vi "Pacemaker ASIC Test_Conditon Globals.vi"() -> ()   [LabVIEW 2016]
uses:
  AET/TypeDef/Pacemaker ASIC Test_Relay Status.ctl
  AET/TypeDef/Pacemaker ASIC Test_Function.ctl
  AET/TypeDef/Pacemaker ASIC Test_Relay Which.ctl
  AET/TypeDef/Pacemaker ASIC Test_Register Mark Type.ctl
  step type.ctl
panel:
  in  "Rk_30":dbl=30000.0
  in  "R 12p5X":dbl
  in  "P 100X":dbl
  in  "PV [C]":dbl=37.0
  in  "Rs_Offset":dbl=23700.0
  in  "175k Downlink Vpp[V]":dbl=0.33
  in  "Rk_20":dbl=24222.307131117894
  in  "Step Type Name":T1=["Basic Setting", "Ibat Test", "Ib Trim Test", "Ib Vs Temp Test", "Ib Vs Vbat Test", "Vref Trim Test", "Vref Vs Temp Test", "Vref Vs Vbat Test", "Vref PSR Test", "VregD Trim Test", "VregD Vs Temp Test", "VregD Vs Vbat Test", "VregD Vs Load Test", "VregD PSR Test", "VregA Trim Test", "VregA Vs Temp Test", "VregA Vs Vbat Test", "VregA Vs Load Test", "VregA PSR Test", "Sense OS1 OS2 Trim Test", "Sense Lpf Hpf Trim Test", "Sense IBIPT Trim Test", "Sense Triangle Waveform Gain Vi Test", "Sense Triangle Waveform Gain Gainout Test", "Sense Pace Rejection Low Sensitivity Test", "Sense Pace Rejection High Sensitivity Test", "Sense Idle Noise Test", "Sense Drain Current Test", "Sense PSR Test", "Sense Pos Triangle Waveform Threshold Test", "Sense Neg Triangle Waveform Threshold Test", "Sense Delay Time 1 Test", "Sense Delay Time 2 Test", "Sense Sine2 Sensitivity Curve Test", "Sense After Sense Test", "Sense After Pace Test", "Sense CMRR Test", "Sense Input Impedance Test", "Pace Pump Efficiency Test", "Pace VH Test", "Pace Recharge Voltage Remain Test", "Pace Amp Test", "Pace Amp GB Test", "Pace Amp 200us Test", "Pace Amp 200us Vs Temp Test", "Pace Amp 200us Vs Battery Imp Test", "Pace Amp 200us Vs PW Test", "Pace Amp 200us Vs Rate Test", "Pace Pulse Width Test", "RC32k Trim Test", "RC32k Jitter Test", "RC32k Vs Vbat Test", "RC1p6k Trim Test", "RC1p6k Jitter Test", "RC1p6k Vs Vbat Test", "32k Crystal Input Under Voltage Test", "32k Crystal Turn on Time Test", "32k Crystal Freq Vs Temp Test", "32k Crystal Duty Vs Temp Test", "32k Crystal Freq Vs Vbat Test", "32k Crystal Duty Vs Vbat Test", "32k Crystal Jitter Test", "Por Power Up Test", "Porn VregD Power Up Test", "Por Power Down Test", "Por Nlsd Power Down Test", "Porn VregD Power Down Test", "Por Glitch Test", "Ant Receive Turn On Time Test", "Ant Receive Turn Off Time Test", "Ant Receive Threshold Test", "Ant Send Drain Current Test", "Ant Send Vpp Test", "ADC Dynamic Parameters Test", "ADC Lead Impedance Test", "ReedSwitch Vs Vbat Test", "Battery Load Impedance Test", "Battery Impedance Test", "Digital 1 Test", "ADC Static Parameters Test", "PR Detection Accuracy Test", "PR Detection Drop Voltage Test", "PR Detection PSR Test", "PR Detection Drain Current Test", "PR Detection Idle Noise Test", "PR Detection Deviation Test", "RC32k Clock Switch Test", "Digital 2 Test", "Register Reset", "Set Rst_Ext", "Trim", "ADC VH Test", "Sense Output Unique Test", "BandGap Setpoint Test", "32k Crystal Setpoint Test", "RC32k Input Under Voltage Test", "RC1p6k Input Under Voltage Test", "ADC Battery V1 Test", "ADC EGM Test", "Pace Average Current Test", "Sense Dynamic Performance Test", "Relay Reset", "Power OnOff", "Set 0V", "ADC Battery V2 Test", "Sense Sine Dynamic Range Test", "Sense Triangle Dynamic Range Test", "Check ASIC VVI\n", "pace gb voltage", "Test Done\n", "Step Test\n", "pace gb pluse width", "pace gb pluse frequency", "pace gb pluse interval", "sensitivity threshold", "MRI Threshold  Cal Test", "MRI Threshold Test"]
  in  "T":dbl
  in  "Reg Data":u8 format="%02x"
  in  "Reg Mark":T2=enum."TRIM_BANDGAPV"
  in  "Relay Index0":T3[](array[typedef])=[enum."CrystalOX2", enum."DtoOutput", enum."spiPXIpacePXI", enum."ADCinNC", enum."noloadcurrent", enum."IPGInputZNC", enum."ReedinDo", enum."AntLC", enum."nomeas", enum."RegDCurNC", enum."LoadRNC", enum."CurrentPumpNC", enum."CurrentSenseNC", enum."Anosignor", enum."Vnosignor", enum."bat0w", enum."currentMeas1", enum."currentMeas2", enum."CrystalOX2", enum."CrystalOX2", enum."CrystalOX2", enum."CrystalOX2", enum."CrystalOX2", enum."CrystalOX2", enum."CrystalOX2", enum."CrystalOX2", enum."CrystalOX2", enum."CrystalOX2", enum."CrystalOX2", enum."CrystalOX2", enum."CrystalOX2", enum."CrystalOX2", enum."CrystalOX2", enum."CrystalOX2", enum."CrystalOX2", enum."CrystalOX2", enum."CrystalOX2"]
  in  "Relay Default":T3[](array[typedef])=[enum."CrystalOX2", enum."DtoOutput", enum."spiPXIpacePXI", enum."ADCinNC", enum."noloadcurrent", enum."IPGInputZNC", enum."ReedinDo", enum."AntLC", enum."nomeas", enum."RegDCurNC", enum."LoadRNC", enum."CurrentPumpNC", enum."CurrentSenseNC", enum."Anosig250w", enum."Vnosig250w", enum."bat200w", enum."currentMeas1", enum."currentMeas2"]
  in  "PS [V]":dbl=2.8
  in  "SV [C]":dbl=37.0
  in  "Trim":u8[](array[numeric])=[8, 9, 9, 9, 16, 16, 8, 8, 32, 32, 16, 16, 16, 16, 8, 8] format="%b"
  in  "Command":T4[](array[typedef])=[enum."Basic Setting", enum."Ibat Test", enum."Ib Trim Test", enum."Ib Vs Temp Test", enum."Ib Vs Vbat Test", enum."Vref Trim Test", enum."Vref Vs Temp Test", enum."Vref Vs Vbat Test", enum."Vref PSR Test", enum."VregD Trim Test", enum."VregD Vs Temp Test", enum."VregD Vs Vbat Test", enum."VregD Vs Load Test", enum."VregD PSR Test", enum."VregA Trim Test", enum."VregA Vs Temp Test", enum."VregA Vs Vbat Test", enum."VregA Vs Load Test", enum."VregA PSR Test", enum."Sense OS1 OS2 Trim Test", enum."Sense Lpf Hpf Trim Test", enum."Sense IBIPT Trim Test", enum."Sense Triangle Waveform Gain Vi Test", enum."Sense Triangle Waveform Gain Gainout Test", enum."Sense Pace Rejection Low Sensitivity Test", enum."Sense Pace Rejection High Sensitivity Test", enum."Sense Idle Noise Test", enum."Sense Drain Current Test", enum."Sense PSRR Test", enum."Sense Pos Triangle Waveform Threshold Test", enum."Sense Neg Triangle Waveform Threshold Test", enum."Sense Delay Time 1 Test", enum."Sense Delay Time 2 Test", enum."Sense Sine2 Sensitivity Curve Test", enum."Sense After Sense Test", enum."Sense After Pace Test", enum."Sense CMRR Test", enum."Sense Input Impedance Test", enum."Pace Pump Efficiency Test", enum."Pace VH Test", enum."Pace Recharge Voltage Remain Test", enum."Pace Amp Test", enum."Pace Amp GB Test", enum."Pace Amp 200us Test", enum."Pace Amp 200us Vs Temp Test", enum."Pace Amp 200us Vs Battery Imp Test", enum."Pace Amp 200us Vs PW Test", enum."Pace Amp 200us Vs Rate Test", enum."Pace Pulse Width Test", enum."RC32k Trim Test", enum."RC32k Jitter Test", enum."RC32k Vs Vbat Test", enum."RC1p6k Trim Test", enum."RC1p6k Jitter Test", enum."RC1p6k Vs Vbat Test", enum."32k Crystal Input Under Voltage Test", enum."32k Crystal Turn on Time Test", enum."32k Crystal Freq Vs Temp Test", enum."32k Crystal Duty Vs Temp Test", enum."32k Crystal Freq Vs Vbat Test", enum."32k Crystal Duty Vs Vbat Test", enum."32k Crystal Jitter Test", enum."Por Power Up Test", enum."Porn VregD Power Up Test", enum."Por Power Down Test", enum."Por Nlsd Power Down Test", enum."Porn VregD Power Down Test", enum."Por Glitch Test", enum."Ant Receive Turn On Time Test", enum."Ant Receive Turn Off Time Test", enum."Ant Receive Threshold Test", enum."Ant Send Drain Current Test", enum."Ant Send Vpp Test", enum."ADC Dynamic Parameters Test", enum."ADC Lead Impedance Test", enum."ReedSwitch Vs Vbat Test", enum."Battery Load Impedance Test", enum."Battery Impedance Test", enum."Digital 1 Test", enum."ADC Static Parameters Test", enum."PR Detection Accuracy Test", enum."PR Detection Drop Voltage Test", enum."PR Detection PSR Test", enum."PR Detection Drain Current Test", enum."PR Detection Idle Noise Test", enum."PR Detection Deviation Test", enum."RC32k Clock Switch Test", enum."Digital 2 Test", enum."Register Reset", enum."Set Rst_Ext", enum."Trim", enum."ADC VH Test", enum."Sense Output Unique Test ", enum."BandGap Setpoint Test", enum."32k Crystal Setpoint Test", enum."RC32k Input Under Voltage Test", enum."RC1p6k Input Under Voltage Test", enum."ADC Battery V1 Test", enum."ADC EGM Test", enum."Pace Average Current Test", enum."Sense Dynamic Performance Test", enum."Relay Reset", enum."Power OnOff", enum."Set 0V", enum."ADC Battery V2 Test", enum."Sense Sine Dynamic Range Test ", enum."Sense Triangle Dynamic Range Test ", enum."Check ASIC VVI", enum."pace gb voltage", enum."Step Test", enum."Test Done", enum."pace gb pluse width", enum."pace gb pluse frequency", enum."pace gb pluse interval", enum."sensitivity threshold", enum."MRI Threshold  Cal Test", enum."MRI Threshold Test"]
  in  "SN":string="24A"
  in  "PN":string="MC02"
  in  "Start Time":string="20120605_124732"
  in  "relay status":T5
  in  "Power Attenuate":dbl=2.0
  # "ibp\nibr\nvregd\nvrega\nota_os1\nota_os2\nhpf_A\nlpf_A\nrc32k\nrc1p6k\nibipt_a\notv_os1\notv_os2\nibipt_v\nhpf_V\nlpf_V"
  # "32k Crystal Freq Vs Temp Test\n32k Crystal Duty Vs Temp Test"
  # "1.5.7 起搏幅度测量（国标1）\tPump Leadding Pulse Detail Test\n起搏幅度测量（国标2）\tPump Pacing amplitude2\n起搏幅度测量（200US）\tPump Pacing amplitude3\n起搏幅度-温度\tPump Pacing amplitude -Temp\n起搏幅度-电池内阻\tPump Pacing amplitude - battery\n起搏幅度-起搏脉宽\tPump Pacing amplitude- pulse width\n起搏幅度-起搏频率\tPump Pacing amplitude -Frequency"
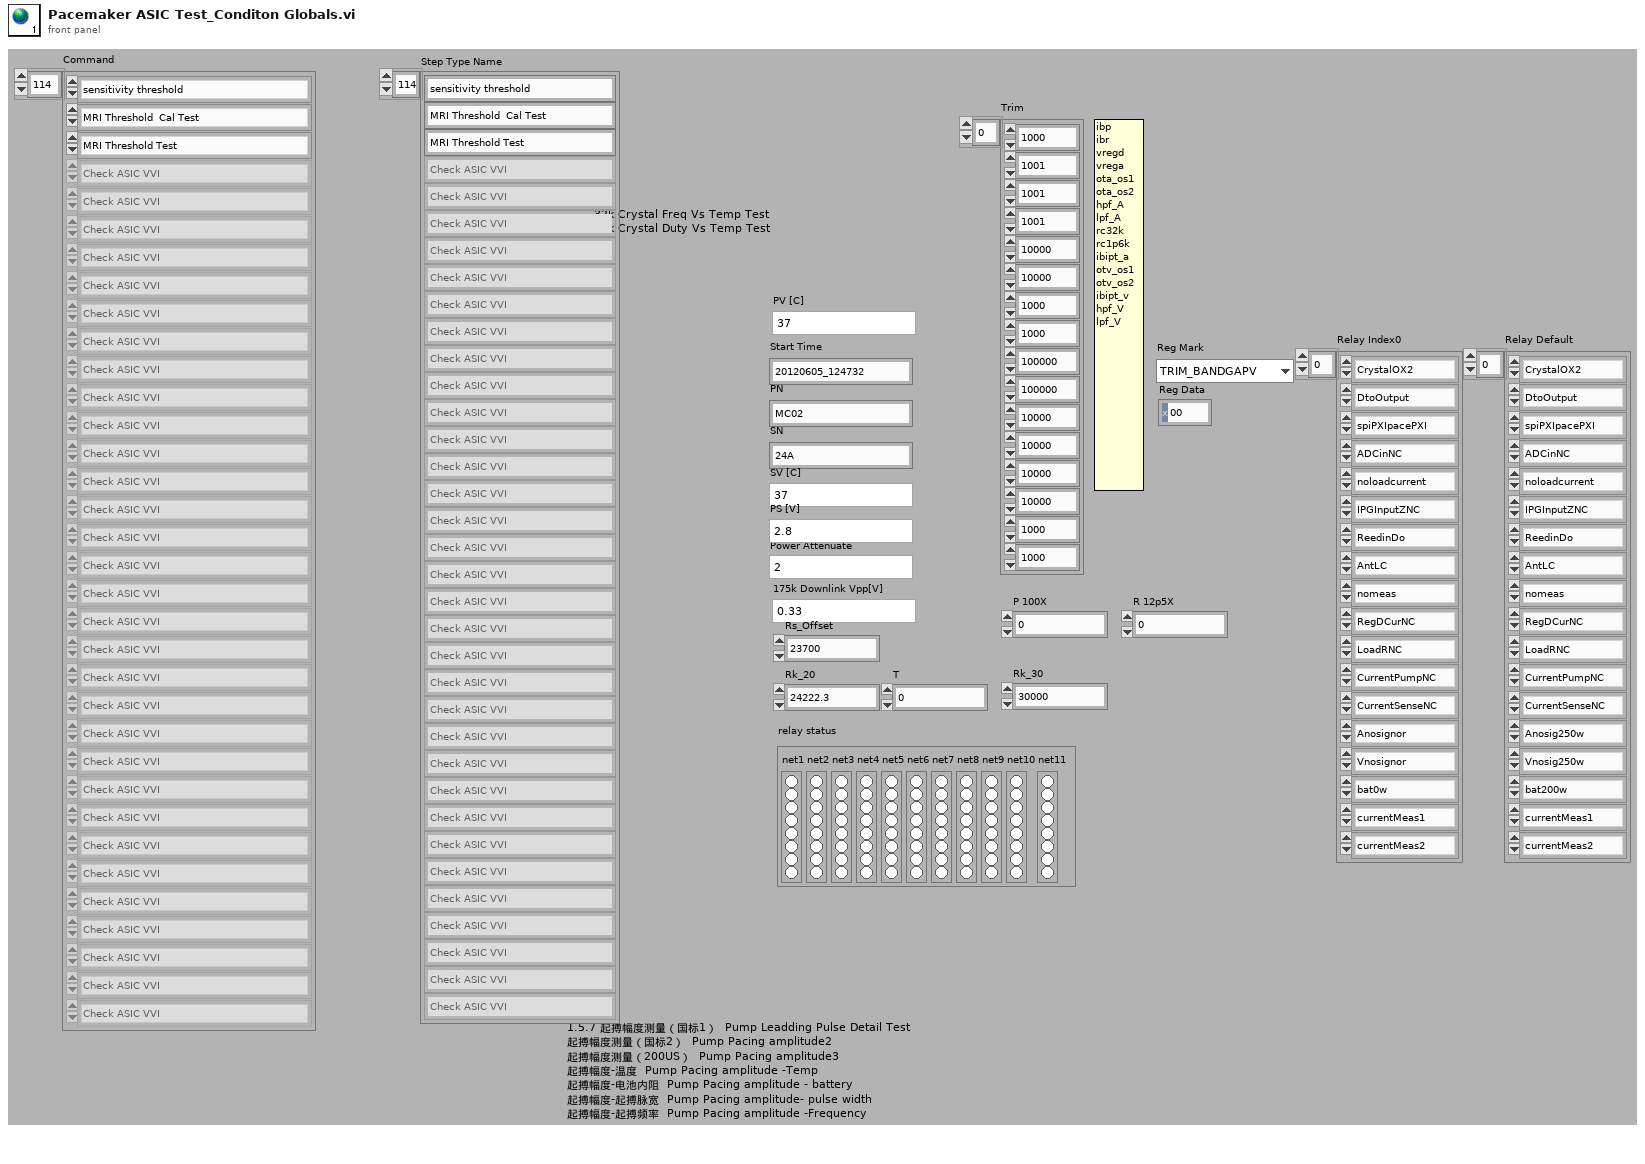
[diagram p1: front panel]
types:
  T1 = typedef "step type.ctl" = string[]
  T2 = typedef "Pacemaker ASIC Test_Register Mark Type.ctl" = enum16{"no action", "TRIM_BANDGAPV", "TRIM_VREGD", "TRIM_VREGA", "TRIM_IBIAS", "TRIM_HPFBW", "TRIM_LPFBW", "TRIM_RC32k", "TRIM_RC1p6k", "TRIM_IBIPT_A", "TRIM_IBIPT_V", "ASGN", "AS", "AUR_UT", "APAMP", "APW", "APUMPGN", "ARCHG", "ABILUNISEL", "VSGN", "VS", "VUR_UT", "VPAMP", "VPW", "VPUMPGN", "VRCHG", "VBILUNISEL", "Test_sel_a", "Test_sel_b", "DTO_SEL", "FBCMEN", "CPEN", "RC1p6kEN", "AntDTM", "ANTENN", "EGMFS REQ", "RC32kEN", "CPUOK", "ENOBLP1", "ENOBLP2", "OBLANK", "PDSA1", "PDSV1", "CSAEN", "CSVEN", "BIR RL", "BIR RH", "MREQ", "RK_SEL", "MRESULT1", "MRESULT2", "TrimOTA_0S1", "TrimOTA_0S2", "TrimOTV_0S1", "TrimOTV_0S2", "ENCASES", "TRIM_HPFBW_H_A", "TRIM_HPFBW_L_A", "TRIM_LPFBW_A", "TRIM_HPFBW_H_V", "TRIM_HPFBW_L_V", "TRIM_LPFBW_V", "R_C_Sel", "PDCHG", "ASIC VVI"}
  T3 = typedef "Pacemaker ASIC Test_Relay Which.ctl" = enum16{"CrystalOX2", "PatternOX2", "DtoOutput", "DtoInput", "spiEM1pacePXI", "spiPXIpacePXI", "ADCinNC", "ADCinAnalog", "noloadcurrent", "curvrega", "curvha", "curvhv", "curvregd", "IPGInputZNC", "IPGringAtipAClose", "IPGringAtipAOpen", "IPGringVtipVClose", "IPGringvtipVOpen", "IPGCasetipAClose", "IPGCasetipAOpen", "IPGCasetipVClose", "IPGCasetipVOpen", "ReedinDo", "ReedinAo", "AntLC", "AntAnalog", "AntDigital", "nomeas", "tennaMeas", "RegDCurNC", "RegDCurMeas", "LoadRNC", "LoadRMeas", "CurrentPumpNC", "CurrentPumpMeas", "CurrentSenseNC", "CurrentSenseMeas", "Anosignor", "Anosig100w", "Anosig250w", "Anosig500w", "Anosig1000w", "Aatte5bip", "Aatte10bip", "Aatte20bip", "Aatte50bip", "Aatte10unip", "Aatte20unip", "Aatte40unip", "Aatte100unip", "Agnd", "Anoatte", "AnoatteCom", "Vnosignor", "Vnosig100w", "Vnosig250w", "Vnosig500w", "Vnosig1000w", "Vatte5bip", "Vatte10bip", "Vatte20bip", "Vatte50bip", "Vatte10unip", "Vatte20unip", "Vatte40unip", "Vatte100unip", "Vgnd", "Vnoatte", "VnoatteCom", "bat0w", "bat200w", "bat500w", "bat1k", "bat5k", "bat10k", "batnocap", "currentMeas1", "currentMeas2"}
  T4 = typedef "Pacemaker ASIC Test_Function.ctl" = enum16{"No Action", "Init", "Init Function", "Close", "Seq Load", "Seq Start", "Relay Reset", "Relay Config", "Register Bit Name Update", "Register Reset", "Register Write", "Register Read", "Register Config", "PCH OnOff", "Trim File Read", "Temp OnOff", "Temp Set", "Temp Check", "Temp Read", "Power OnOff", "Set 0V", "Create DAQmx Task", "Set TestMode", "Set Rst_Ext", "AI Task", "Basic Setting", "Ibat Test", "Ib Trim Test", "Ib Vs Temp Test", "Ib Vs Vbat Test", "Vref Trim Test", "Vref Vs Temp Test", "Vref Vs Vbat Test", "Vref PSR Test", "VregD Trim Test", "VregD Vs Temp Test", "VregD Vs Vbat Test", "VregD Vs Load Test", "VregD PSR Test", "VregA Trim Test", "VregA Vs Temp Test", "VregA Vs Vbat Test", "VregA Vs Load Test", "VregA PSR Test", "Sense OS1 OS2 Trim Test", "Sense Lpf Hpf Trim Test", "Sense IBIPT Trim Test", "Sense Triangle Waveform Gain Vi Test", "Sense Triangle Waveform Gain Gainout Test", "Sense Pace Rejection Low Sensitivity Test", "Sense Pace Rejection High Sensitivity Test", "Sense Idle Noise Test", "Sense Drain Current Test", "Sense PSRR Test", "Sense Pos Triangle Waveform Threshold Test", "Sense Neg Triangle Waveform Threshold Test", "Sense Delay Time 1 Test", "Sense Delay Time 2 Test", "Sense Sine2 Sensitivity Curve Test", "Sense After Sense Test", "Sense After Pace Test", "Sense CMRR Test", "Sense Input Impedance Test", "Pace Pump Efficiency Test", "Pace VH Test", "Pace Recharge Voltage Remain Test", "Pace Amp Test", "Pace Amp GB Test", "Pace Amp 200us Test", "Pace Amp 200us Vs Temp Test", "Pace Amp 200us Vs Battery Imp Test", "Pace Amp 200us Vs PW Test", "Pace Amp 200us Vs Rate Test", "Pace Pulse Width Test", "RC32k Trim Test", "RC32k Jitter Test", "RC32k Vs Vbat Test", "RC32k Clock Switch Test", "RC1p6k Trim Test", "RC1p6k Jitter Test", "RC1p6k Vs Vbat Test", "32k Crystal Input Under Voltage Test", "32k Crystal Turn on Time Test", "32k Crystal Freq Vs Temp Test", "32k Crystal Duty Vs Temp Test", "32k Crystal Freq Vs Vbat Test", "32k Crystal Duty Vs Vbat Test", "32k Crystal Jitter Test", "Por Power Up Test", "Porn VregD Power Up Test", "Por Power Down Test", "Por Nlsd Power Down Test", "Porn VregD Power Down Test", "Por Glitch Test", "Ant Receive Turn On Time Test", "Ant Receive Turn Off Time Test", "Ant Receive Threshold Test", "Ant Send Drain Current Test", "Ant Send Vpp Test", "ADC Dynamic Parameters Test", "ADC Lead Impedance Test", "ReedSwitch Vs Vbat Test", "Battery Load Impedance Test", "Battery Impedance Test", "Digital 1 Test", "ADC Static Parameters Test", "Trim", "PR Detection Accuracy Test", "PR Detection Drop Voltage Test", "PR Detection PSR Test", "PR Detection Drain Current Test", "PR Detection Idle Noise Test", "PR Detection Deviation Test", "Digital 2 Test", "ADC VH Test", "Sense Output Unique Test ", "BandGap Setpoint Test", "32k Crystal Setpoint Test", "Stop Temp", "RC32k Input Under Voltage Test", "RC1p6k Input Under Voltage Test", "ADC Battery V1 Test", "ADC EGM Test", "Pace Average Current Test", "Sense Dynamic Performance Test", "ADC Battery V2 Test", "Sense Sine Dynamic Range Test ", "Sense Triangle Dynamic Range Test ", "Check ASIC VVI", "pace gb voltage", "Test Done", "Step Test", "pace gb pluse width", "pace gb pluse frequency", "pace gb pluse interval", "sensitivity threshold", "MRI Threshold  Cal Test", "MRI Threshold Test"}
  T5 = typedef "Pacemaker ASIC Test_Relay Status.ctl" = cluster{"net1":bool[], "net2":bool[], "net3":bool[], "net4":bool[], "net5":bool[], "net6":bool[], "net7":bool[], "net8":bool[], "net9":bool[], "net10":bool[], "net11":bool[]}
diagram:
